vi "Build Ymodem First  or End Frame.vi"(9 "File Size(KB)":dbl, 10 "File Name":string, 11 "Mode(First Frame)":enum16{"First Frame", "End Frame"}(ring)) -> (1 "File Size(Byte)":u32 format="%.0x", 3 "Frame Data":u8[](array[numeric]) format="%02x")   [LabVIEW 2013]
doc: "Build the data frame(header part or end part) for the YModem protocol."
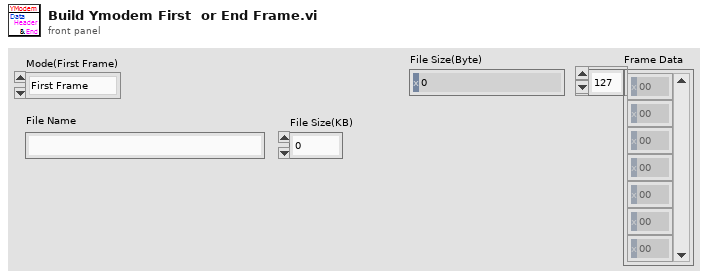
[diagram p1: front panel]
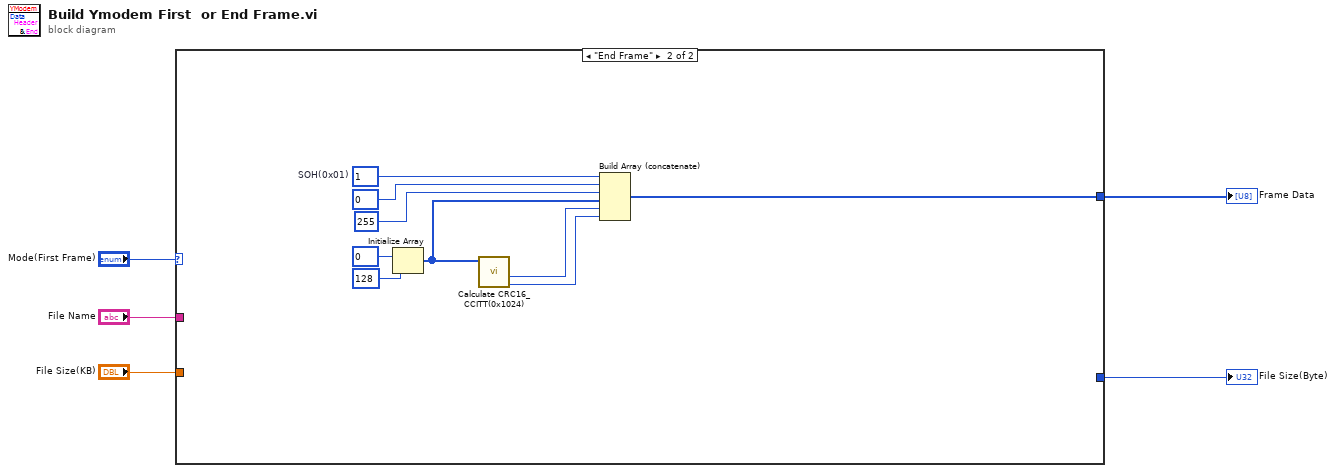
[diagram p0: block diagram]
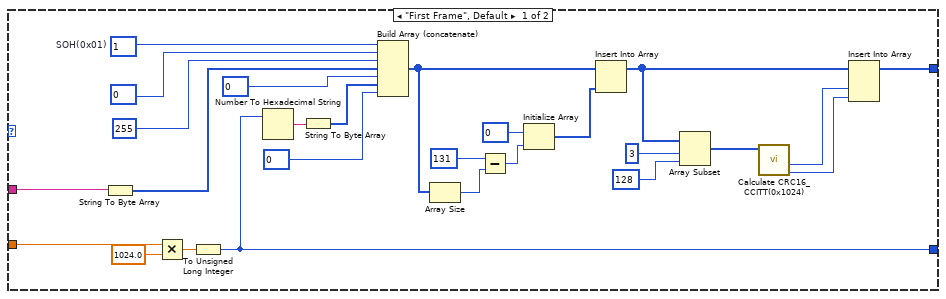
[diagram p2: hidden frame]
diagram:
  n1 = case shown="\"End Frame\"" "Mode(First Frame)" {
    tunnel: "File Size(KB)" -> [w31 _]
    tunnel: "File Name" -> [w27 _]
    tunnel: [w26 _] -> w3
    tunnel: [w12 w35] -> w2
    frame "First Frame", Default {
      w8 = u8 1  # SOH(0x01)
      n2 = String To Byte Array(string=w27) -> (unsigned byte array=w24:u8[])
      n3 = Multiply(x=w31, y=1024.0) -> (x*y=w30:dbl)
      n4 = To Unsigned Long Integer(number=w30) -> (unsigned 32bit integer=w26:u32)
      n5 = Number To Hexadecimal String(2:w26) -> (0:w25:string)  [unwired: 1 in]
      n6 = String To Byte Array(string=w25) -> (unsigned byte array=w22:u8[])
      n7 = Build Array (concatenate)(w8, u8 0 ("Numeric"), u8 255 ("Numeric"), w24, u8 0 ("Numeric"), w22, u8 0 ("Numeric")) -> (w17:u8[])
      n8 = Array Size(array=w17) -> (size(s)=w19:i32)
      n9 = Subtract(x=131 ("dimension size"), y=w19) -> (x-y=w18:i32)
      n10 = Initialize Array(u8 0 ("Numeric"), w18) -> (w16:u8[])
      n11 = Insert Into Array(array=w17, new element=w16) -> (w15:u8[])  [unwired: 1 in]
      n12 = Array Subset(array=w15, index=3, length=128) -> (w11:u8[])
      n13 = call "Calculate CRC16_CCITT(0x1024).vi"("Data in"=w11) -> ("Lo CRC16"=w9:u8, "Hi CRC16"=w10:u8)  [unwired: 7 in, 2 out]
      n14 = Insert Into Array(array=w15, new element #1=w10, new element #2=w9) -> (w12:u8[])  [unwired: 1 in]
    }
    frame "End Frame" {
      w40 = u8 1  # SOH(0x01)
      n15 = Initialize Array(u8 0 ("Numeric"), 128 ("dimension size")) -> (w34:u8[])
      n16 = call "Calculate CRC16_CCITT(0x1024).vi"("Data in"=w34) -> ("Lo CRC16"=w32:u8, "Hi CRC16"=w33:u8)  [unwired: 7 in, 2 out]
      n17 = Build Array (concatenate)(w40, u8 0 ("Numeric"), u8 255 ("Numeric"), w34, w33, w32) -> (w35:u8[])
    }
  }
  "File Size(Byte)" <- w3
  "Frame Data" <- w2
